vi "CfgManager.Text.INI (NumericArray) Test Launcher.vi"() -> ()   [LabVIEW 2013]
uses:
  source/Manager.Text.INI/ConfigManager.Text.INI.lvclass
  source/Manager/ConfigManager.lvclass
panel:
  out "data":dbl[](array[numeric])
  out "Keys":string[](array[string])
  out "error out":errorcluster
  out "filepath":path
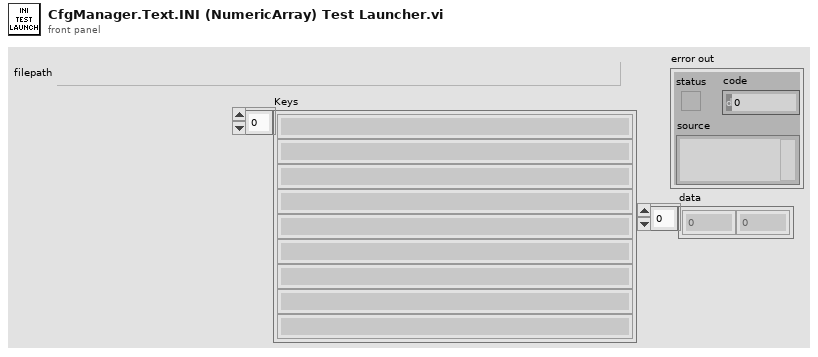
[diagram p1: front panel]
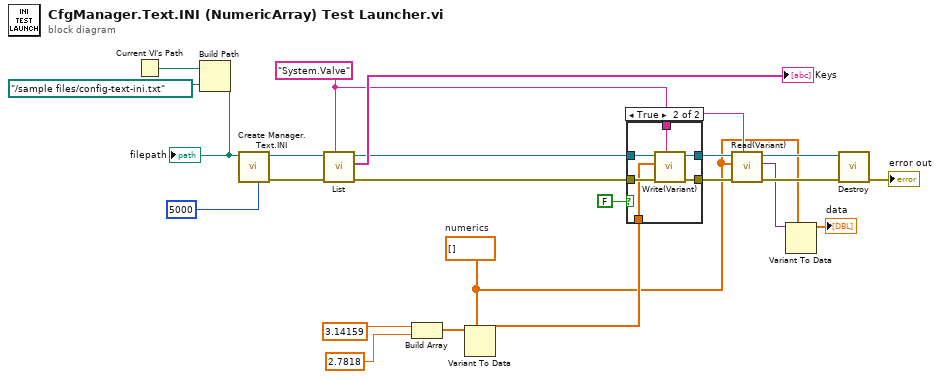
[diagram p0: block diagram]
diagram:
  w4 = dbl[] []  # numerics
  w5 = "System.Valve" ("Qualified Name")
  n1 = Current VI's Path() -> (path=w21:path)
  n2 = Build Path(base path=w21, name or relative path=path "../sample files/config-text-ini.txt" ("filepath 2")) -> (appended path=w19:path)
  "filepath" <- w19
  n3 = call "Create Manager.Text.INI.vi"("write delay (ms)"=5000, "filepath"=w19) -> ("error out"=w17:errorcluster, "ConfigManager.Text.INI out"=w18:refnum<class "ConfigManager.Text.INI.lvclass">)  [unwired: 7 in, 1 out]
  n4 = call "List.vi"("Qualified Name"=w5, "error in (no error)"=w17, "ConfigManager in"=w18) -> ("error out"=w6:errorcluster, "Keys"=→"Keys":string[], "ConfigManager out"=w7:refnum<class "ConfigManager.Text.INI.lvclass">)  [unwired: 6 in]
  n5 = Build Array(3.14159 ("Sensor"), 2.7818 ("Sensor")) -> (w15:dbl[])
  n6 = Variant To Data(type=w4, Variant=w15) -> (data=w14:dbl[])  [unwired: 1 in, 1 out]
  n7 = case shown="True" FALSE {
    tunnel: w7 -> [w25 w31]
    tunnel: w6 -> [w24 w30]
    tunnel: w14 -> [_ w29]
    tunnel: [w25 w28] -> w13
    tunnel: [w24 w27] -> w11
    tunnel: w5 -> [_ w26]
    frame False {
    }
    frame True {
      n8 = call "Write(Variant).vi"("Qualified Name"=w26, "error in (no error)"=w30, "value"=w29, "ConfigManager in"=w31) -> ("error out"=w27:errorcluster, "ConfigManager out"=w28:refnum<class "ConfigManager.Text.INI.lvclass">)  [unwired: 5 in, 1 out]
    }
  }
  n9 = call "Read(Variant).vi"("Qualified Name"=w5, "error in (no error)"=w11, "Type"=w4, "ConfigManager in"=w13) -> ("error out"=w10:errorcluster, "value"=w9:variant, "ConfigManager out"=w12:refnum<class "ConfigManager.Text.INI.lvclass">)  [unwired: 3 in, 2 out]
  n10 = Variant To Data(type=w4, Variant=w9) -> (data=→"data":dbl[])  [unwired: 1 in, 1 out]
  n11 = call-dynamic "Destroy.vi"("error in (no error)"=w10, "ConfigManager.Text in"=w12) -> ("error out"=→"error out":errorcluster)  [unwired: 8 in, 1 out]
